vi "check_mio.vi"() -> ()   [LabVIEW 2013]
uses:
  <vilib>/DAQmx/write.llb/DAQmx Write (Analog Wfm 1Chan NSamp).vi
  <vilib>/DAQmx/create/channels.llb/DAQmx Create Channel (AO-Voltage-Basic).vi
  <vilib>/DAQmx/configure/timing.llb/DAQmx Timing (Use Waveform).vi
  <vilib>/DAQmx/miscellaneous.llb/DAQmx Fill In Error Info.vi
panel:
  out "1/x":dbl
  out "number of samples written per channel":u32
  out "x/y":dbl
  out "output waveform":waveform(dbl)
  out "Waveform Graph":waveform(dbl)(graph)
  in  "Exit":bool
  in  "T":dbl=1.0
  in  "N_steps_1":i32=500 min=0 step=1
  out "DAC_status":bool
  in  "DAC channel":tag="Dev1/ao0"
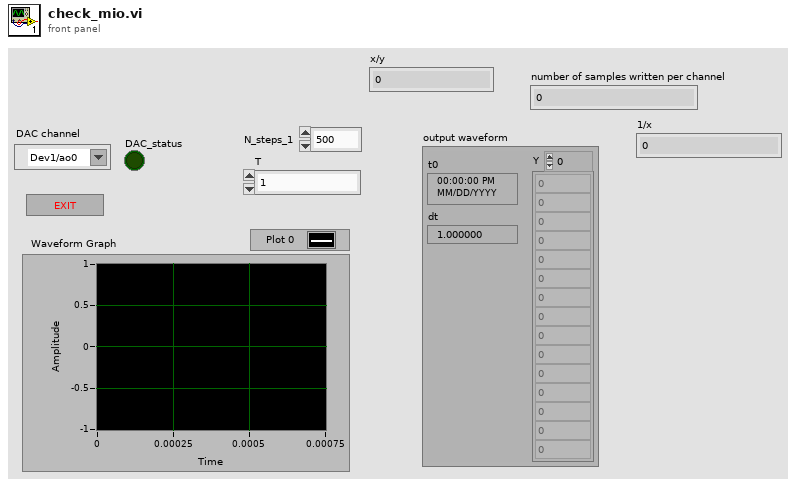
[diagram p1: front panel]
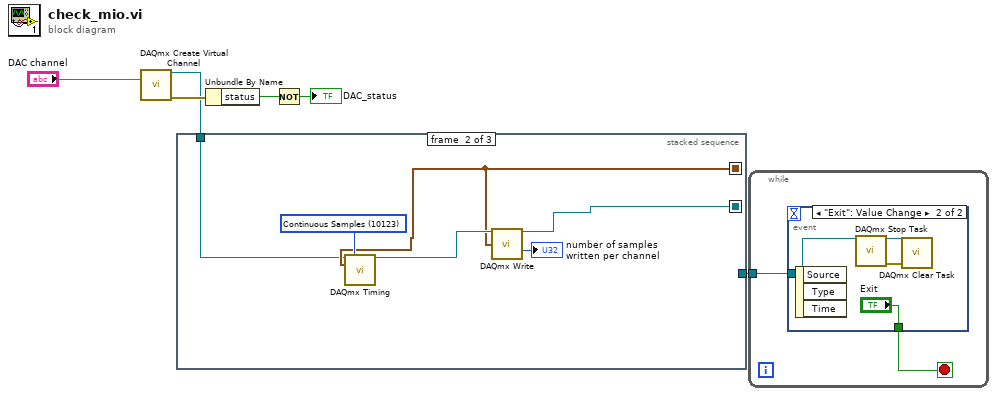
[diagram p0: block diagram]
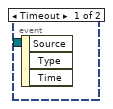
[diagram p2: hidden frame]
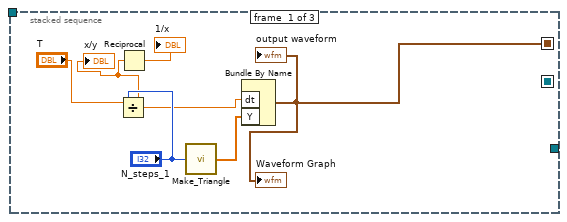
[diagram p3: hidden frame]
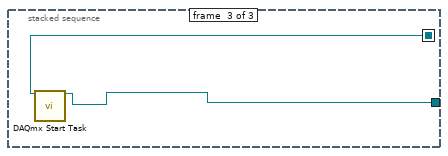
[diagram p4: hidden frame]
diagram:
  n1 = call-poly <vilib>:"DAQmx Create Virtual Channel.vi"("physical channels"="DAC channel") -> ("task out"=w2:refnum<k21>, "error out"=w5:errorcluster)  [unwired: 13 in]
  n2 = stacked-sequence {
    seq-local: [w9 _ _] -> [_ w16 _]
    seq-local: [_ w14 _] -> [_ _ w20]
    tunnel: w2 -> [_ w15 _]
    tunnel: [_ _ w19] -> w1
    frame #0 {
      n3 = Divide(x="T", y="N_steps_1") -> (x/y=w8:dbl)
      "x/y" <- w8
      n4 = Reciprocal(x=w8) -> (1/x=→"1/x":dbl)
      n5 = call "Make_Triangle.vi"("N_steps_1"="N_steps_1") -> ("TriangleWaveform"=w11:dbl[])
      n6 = Bundle By Name("dt"=w8, "Y"=w11) -> (w9:waveform(dbl))  [unwired: 1 in]
      "Waveform Graph" <- w9
      "output waveform" <- w9
    }
    frame #1 {
      w17 = 10123 items=["Finite Samples"=10178, "Continuous Samples"=10123, "Hardware Timed Single Point"=12522] ("sample mode")
      n7 = call-poly <vilib>:"DAQmx Timing.vi"("task/channels in"=w15, "sample mode"=w17, "waveform"=w16) -> ("task out"=w18:refnum<k21>)  [unwired: 11 in, 1 out]
      n8 = call-poly <vilib>:"DAQmx Write.vi"("task/channels in"=w18, "data"=w16) -> ("task out"=w14:refnum<k21>, "number of samples written per channel"=→"number of samples written per channel":u32)  [unwired: 11 in, 1 out]
    }
    frame #2 {
      n9 = call <vilib>:"DAQmx Start Task.vi"("task/channels in"=w20) -> ("task out"=w19:refnum<k21>)  [unwired: 13 in, 1 out]
    }
  }
  n10 = Unbundle By Name(w5) -> ("status"=w4:bool)
  n11 = Not(x=w4) -> (.not. x?=→"DAC_status":bool)
  n12 = while {
    tunnel: w1 -> [w22]
    stop <- w21 stop-if-true
    n13 = event shown="[1] \"Exit\": Value Change" {
      selector: _ -> [_ _]
      dyn-events: _ -> [_ _]
      timeout: _ -> [_ _]
      tunnel: w22 -> [_ w26]
      tunnel: [_ "Exit"] -> w21
      event Timeout {
        n14 = event-data() -> ()  [unwired: 1 in, 3 out]
      }
      event "Exit": Value Change {
        n15 = event-data() -> ()  [unwired: 1 in, 3 out]
        n16 = call <vilib>:"DAQmx Stop Task.vi"("task/channels in"=w26) -> ("task out"=w24:refnum<k21>, "error out"=w23:errorcluster)  [unwired: 13 in]
        n17 = call <vilib>:"DAQmx Clear Task.vi"("task in"=w24, "error in"=w23) -> ()  [unwired: 13 in, 1 out]
      }
    }
  }
